vi "Control Loop_Main.vi"(8 "error in (no error)":errorcluster, 11 "Main Process Class In":refnum<class "Main Class.lvclass">) -> ()   [LabVIEW 2019]
uses:
  Class/Main Process Class/Main Class.lvclass
  LLB/Commonly VI/Main Glb.vi
  LLB/Commonly VI.lvlib
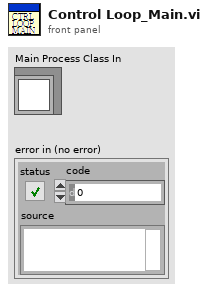
[diagram p1: front panel]
types:
  T1 = typedef "Control Loop_Control.ctl" = enum16{"Initial", "Standby Mode", "Run Mode", "Status", "Exit"}
  T2 = typedef "Control Loop_Status.ctl" = enum16{"None", "Next", "Error", "SafeDoor", "Exit"}
  T3 = cluster{"Control":T1, "Status":T2, "Name":string, "error":errorcluster}
  T4 = cluster{"AutoRunFlg":refnum<vi>, "Action Finish Flg":refnum<vi>, "Remaining Action":refnum<vi>, "Btn_AutoRun":refnum<vi>, "Manual Flg":refnum<vi>, "Sub Process Error":refnum<vi>}
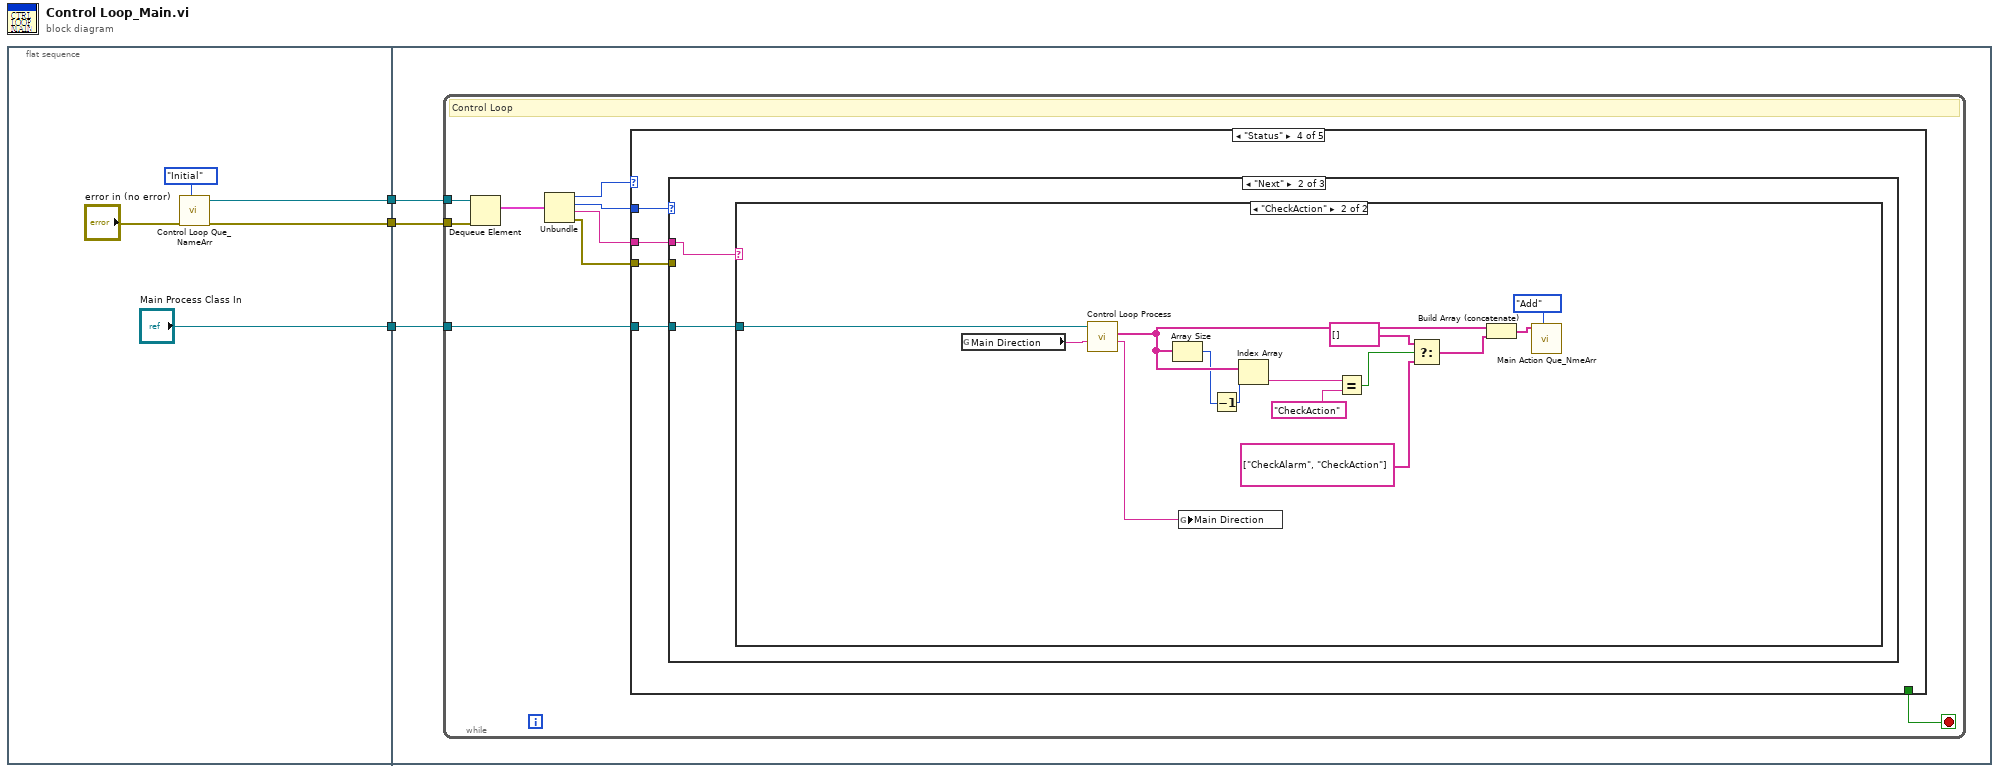
[diagram p0: block diagram]
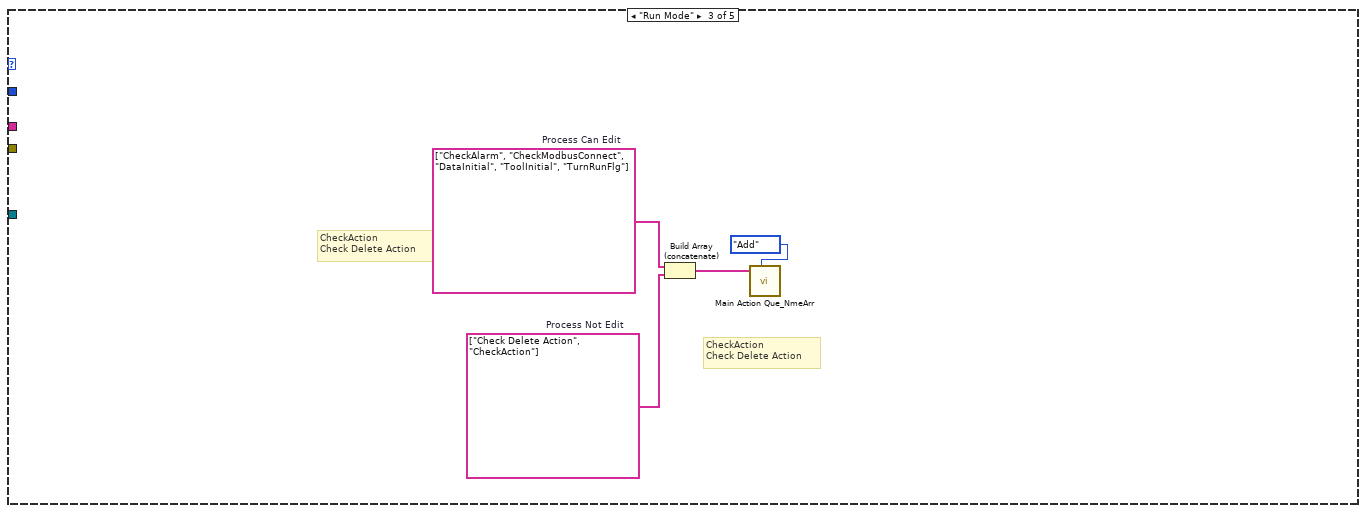
[diagram p4: hidden frame]
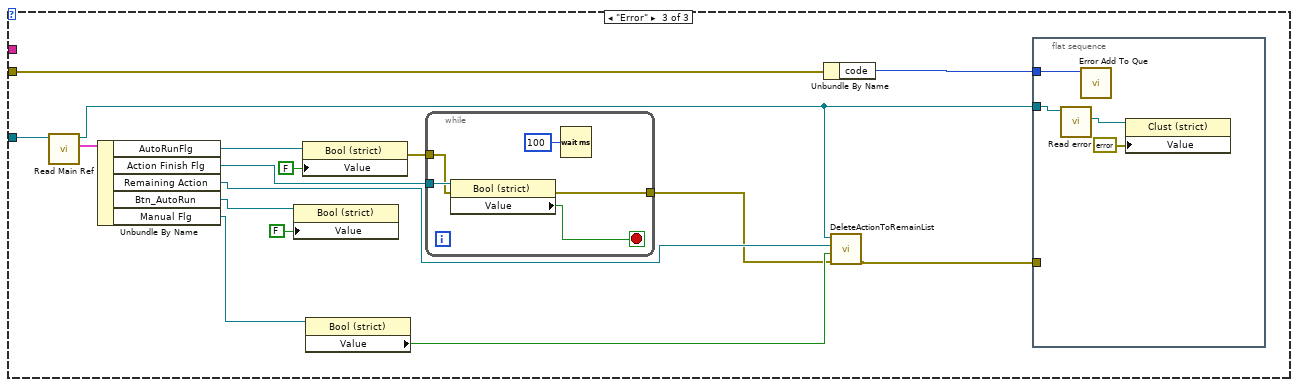
[diagram p7: hidden frame]
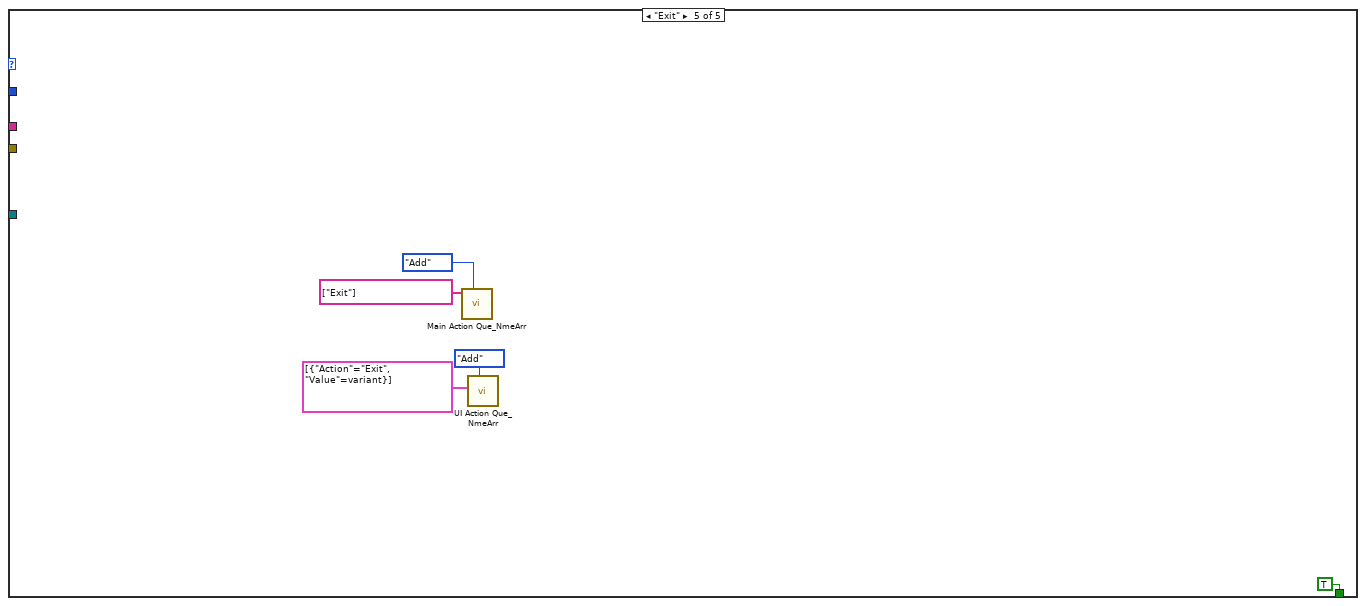
[diagram p8: hidden frame]
diagram:
  n1 = flat-sequence {
    tunnel: [w7] -> w3
    tunnel: [w5] -> w2
    tunnel: ["Main Process Class In"] -> w1
    tunnel: w3 -> [w11]
    tunnel: w2 -> [w10]
    tunnel: w1 -> [w9]
    frame #0 {
      n2 = call "Control Loop Que_NameArr.vi"("Action Select"=enum16{"Initial", "Add", "Release"}."Initial", "error in (no error)"="error in (no error)") -> ("error out"=w7:errorcluster, "Control Loop Q Out"=w5:refnum<queue>)  [unwired: 8 in]
    }
    frame #1 {
      n3 = while {
        tunnel: w11 -> [w14]
        tunnel: w10 -> [w13]
        tunnel: w9 -> [w12]
        stop <- w16 stop-if-true
        # "Control Loop"
        n4 = Dequeue Element(queue=w13, error in (no error)=w14) -> (element=w17:T3)  [unwired: 1 in, 3 out]
        n5 = Unbundle(w17) -> ("Control"=w20:T1, "Status"=w19:T2, "Name"=w18:string, "error"=w15:errorcluster)
        n6 = case shown="\"Status\"" w20 {
          tunnel: w19 -> [_ _ _ w28 _]
          tunnel: w18 -> [_ _ _ w27 _]
          tunnel: [_ _ _ _ TRUE] -> w16
          tunnel: w15 -> [_ _ _ w26 _]
          tunnel: w12 -> [_ _ _ w25 _]
          frame "Initial", Default {
          }
          frame "Standby Mode" {
          }
          frame "Run Mode" {
            w21 = string[] ["Check Delete Action", "CheckAction"]  # Process Not Edit
            w22 = string[] ["CheckAlarm", "CheckModbusConnect", "DataInitial", "ToolInitial", "TurnRunFlg"]  # Process Can Edit
            # "CheckAction\nCheck Delete Action"
            # "CheckAction\nCheck Delete Action"
            n7 = Build Array (concatenate)(w22, w21) -> (w23:string[])
            n8 = call "Main Action Que_NmeArr.vi"("Action"=enum16{"Initial", "Add", "Release"}."Add", "Process"=w23) -> ()  [unwired: 8 in, 2 out]
          }
          frame "Status" {
            n9 = case shown="\"Next\"" w28 {
              tunnel: w27 -> [_ w30 _]
              tunnel: w26 -> [_ _ w56]
              tunnel: w25 -> [_ w29 w60]
              frame "None", Default {
              }
              frame "Next" {
                n10 = case shown="\"CheckAction\"" w30 {
                  tunnel: w29 -> [_ w44]
                  frame "None", Default {
                  }
                  frame "CheckAction" {
                    n11 = global read "Main Glb.vi" "Main Direction"() -> (w32:string)
                    n12 = call-dynamic "Control Loop Process.vi"("MainDirectionIn"=w32, "Main Process Class in"=w44) -> ("MainDirectionOut"=w31:string, "ProcessAction"=w41:string[])  [unwired: 6 in, 2 out]
                    n13 = Array Size(array=w41) -> (size(s)=w40:i32)
                    n14 = global write "Main Glb.vi" "Main Direction"(w31) -> ()
                    n15 = Decrement(x=w40) -> (x-1=w39:i32)
                    n16 = Index Array(array=w41, index=w39) -> (element=w38:string)
                    n17 = Equal?(x=w38, y="CheckAction") -> (x = y?=w36:bool)
                    n18 = Select(t=string[] [], s=w36, f=string[] ["CheckAlarm", "CheckAction"]) -> (s? t:f=w42:string[])
                    n19 = Build Array (concatenate)(w41, w42) -> (w33:string[])
                    n20 = call "Main Action Que_NmeArr.vi"("Action"=enum16{"Initial", "Add", "Release"}."Add", "Process"=w33) -> ()  [unwired: 8 in, 2 out]
                  }
                }
              }
              frame "Error" {
                n21 = call-dynamic "Read Main Ref.vi"("Main Process Class in"=w60) -> ("Main Ref"=w59:T4, "Main Process Class out"=w47:refnum<class "Main Class.lvclass">)  [unwired: 8 in, 1 out]
                n22 = Unbundle By Name(w59) -> ("AutoRunFlg"=w58:refnum<vi>, "Action Finish Flg"=w55:refnum<vi>, "Remaining Action"=w48:refnum<vi>, "Btn_AutoRun"=w51:refnum<vi>, "Manual Flg"=w50:refnum<vi>)
                n23 = property class="Bool (strict)"(reference=w51, "Value"=FALSE) -> ()  [unwired: 1 in, 2 out]
                n24 = property class="Bool (strict)"(reference=w58, "Value"=FALSE) -> (error out=w54:errorcluster)  [unwired: 1 in, 1 out]
                n25 = property class="Bool (strict)"(reference=w50) -> ("Value"=w49:bool)  [unwired: 1 in, 2 out]
                n26 = while {
                  tunnel: w55 -> [w69]
                  tunnel: w54 -> [w66]
                  tunnel: [w65] -> w45
                  stop <- w67 stop-if-true
                  n27 = property class="Bool (strict)"(reference=w69, error in=w66) -> (error out=w65:errorcluster, "Value"=w67:bool)  [unwired: 1 out]
                  n28 = Wait (ms)(milliseconds to wait=u32 100) -> ()  [unwired: 1 out]
                }
                n29 = Unbundle By Name(w56) -> ("code"=w53:i32)
                n30 = call-dynamic "DeleteActionToRemainList.vi"("error in (no error)"=w45, "ManualFlg"=w49, "Remaining Action"=w48, "Main Class in"=w47) -> ("error out"=w46:errorcluster)  [unwired: 6 in, 1 out]
                n31 = flat-sequence {
                  tunnel: w46 -> [_]
                  tunnel: w53 -> [w64]
                  tunnel: w47 -> [w63]
                  frame #0 {
                    n32 = call-dynamic "Read error.vi"("Main Class in"=w63) -> ("error"=w62:refnum<vi>)  [unwired: 8 in, 2 out]
                    n33 = call "Error Add To Que.vi"("Error Code"=w64) -> ()  [unwired: 11 in]
                    n34 = property class="Clust (strict)"(reference=w62, "Value"=errorcluster {"status"=FALSE, "code"=0, "source"=""}) -> ()  [unwired: 1 in, 2 out]
                  }
                }
              }
            }
          }
          frame "Exit" {
            n35 = call "Main Action Que_NmeArr.vi"("Action"=enum16{"Initial", "Add", "Release"}."Add", "Process"=string[] ["Exit"]) -> ()  [unwired: 8 in, 2 out]
            n36 = call "UI Action Que_NmeArr.vi"("Action"=enum16{"Initial", "Add", "Release"}."Add", "UI Process"=cluster{"Action":string, "Value":variant}[] [{"Action"="Exit", "Value"=variant}]) -> ()  [unwired: 8 in, 2 out]
          }
        }
      }
    }
  }
